vi "parser.vi"() -> ()   [LabVIEW 2013]
panel:
  out "x .and. y?":u8
  out "String":string
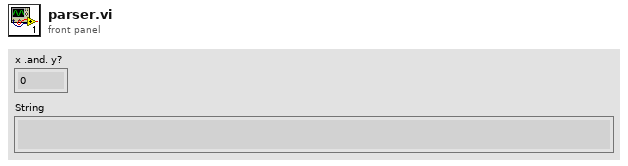
[diagram p1: front panel]
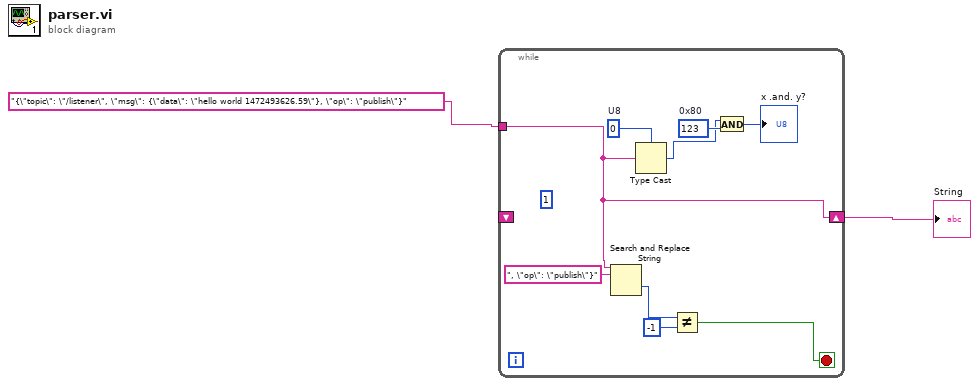
[diagram p0: block diagram]
diagram:
  n1 = while {
    shift-right: [w4] -> w1
    shift-left: _ -> [_]
    tunnel: "{\"topic\": \"/listener\", \"msg\": {\"data\": \"hello world 1472493626.59\"}, \"op\": \"publish\"}" -> [w4]
    stop <- w5 stop-if-true
    w10 = u8 123  # 0x80
    w11 = u8 0  # U8
    (unwired) 1 ("bytes to read")
    n2 = Search and Replace String(input string=w4, search string=", \"op\": \"publish\"}") -> (offset past replacement=w7:i32)  [unwired: 6 in, 3 out]
    n3 = Type Cast(type=w11, x=w4) -> (*(type *) &x=w9:u8)
    n4 = Not Equal?(x=w7, y=-1) -> (x != y?=w5:bool)
    n5 = And(x=w9, y=w10) -> (x .and. y?=→"x .and. y?":u8)
  }
  "String" <- w1
